vi "Write Parameters.vi"(10 "Parameters":u32[](array[numeric])=[600000, 60000, 100, 3], 11 "valve_VCH_ZM_state in":refnum<class "valve_VCH_ZM_state.lvclass">) -> (3 "valve_VCH_ZM_state out":refnum<class "valve_VCH_ZM_state.lvclass">)   [LabVIEW 2019, in "valve_VCH_ZM_state.lvclass"]
uses:
  valve_VCH_ZM_state.lvclass
  valve_VCH_ZM_state.lvclass/valve_VCH_ZM_state.ctl
panel:
  # "0 - T_big_pause\n1 - T_little_pause\n2 - T_impuls\n3 - N_repeat"
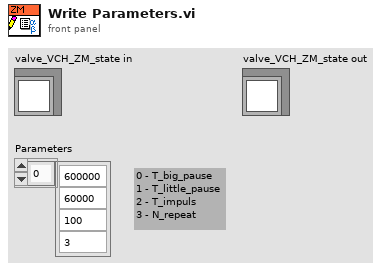
[diagram p1: front panel]
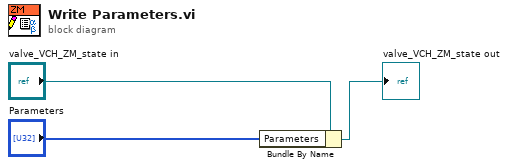
[diagram p0: block diagram]
diagram:
  n1 = Bundle By Name(cluster="valve_VCH_ZM_state in", "Parameters"="Parameters") -> (→"valve_VCH_ZM_state out":refnum<class "valve_VCH_ZM_state.lvclass">)
